vi "Save Instance VI to Polymorphic.vi"(8 "error in (no error)":errorcluster, 9 "Polymorphic Label":string, 10 "SubVI Ref In":refnum<vi>, 11 "Library Ref In":refnum<vi>) -> (0 "error out":errorcluster)   [LabVIEW 2020]
doc: "Duplicates the malleable VI instance to a new VI, and adds the new VI to a polymorphic VI."
uses:
  Global.vi
  <vilib>/LabVIEW Icon API/LabVIEW Icon API.lvlib
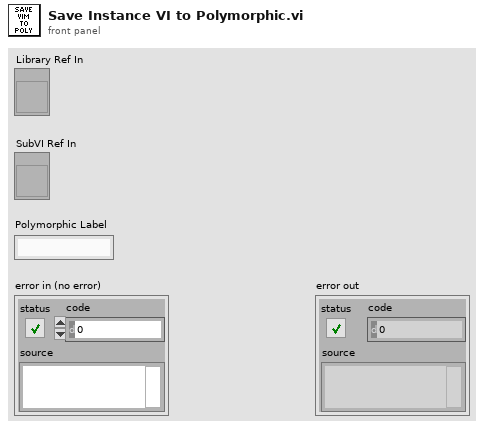
[diagram p1: front panel]
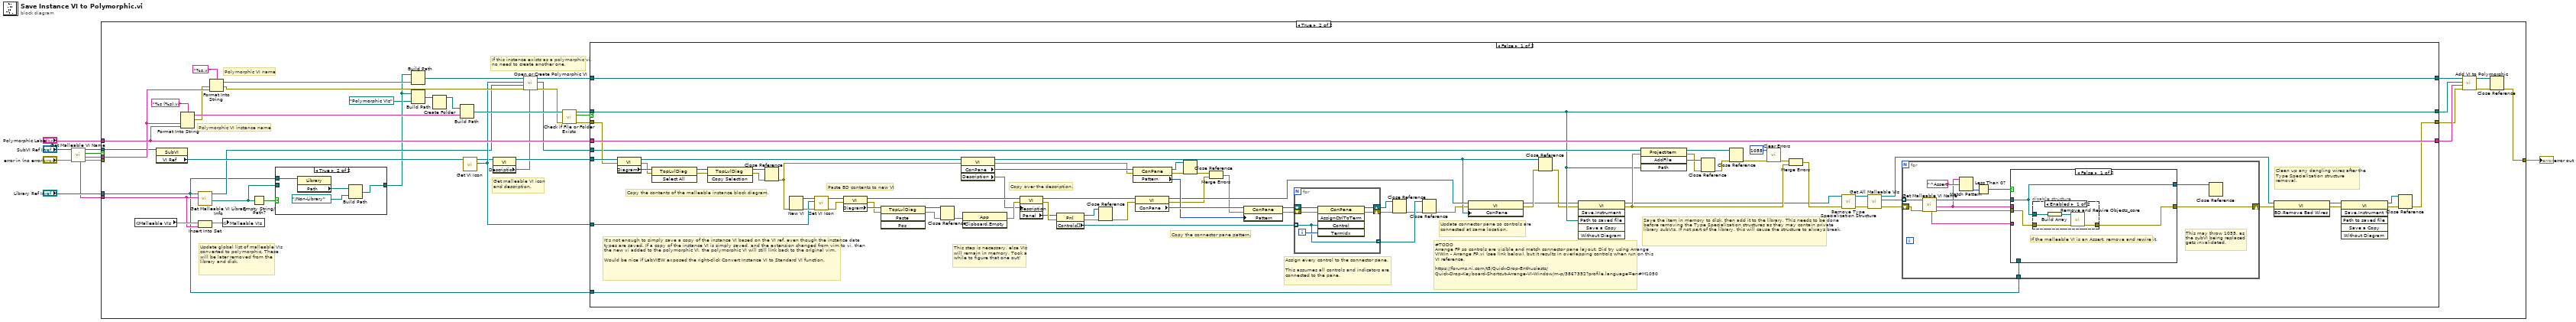
[diagram p0: block diagram]
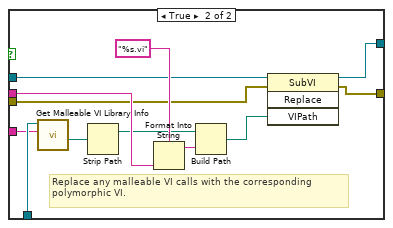
[diagram p4: hidden frame]
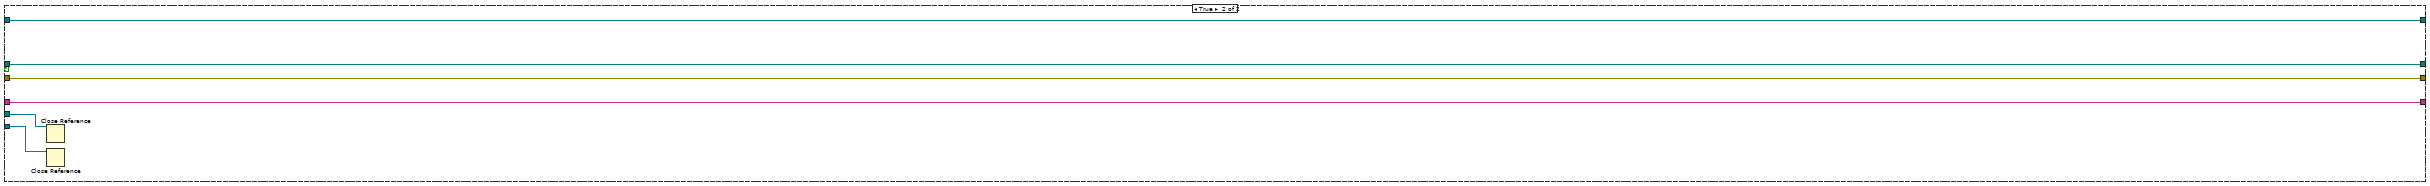
[diagram p5: hidden frame]
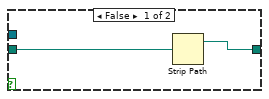
[diagram p6: hidden frame]
diagram:
  n1 = call "Get Malleable VI Name.vi"("error in (no error)"="error in (no error)", "SubVI Ref In"="SubVI Ref In") -> ("error out"=w5:errorcluster, "Name without extension"=w8:string, "Is Malleable VI?"=w1:bool, "SubVI Ref Out"=w9:refnum<vi>, "Name (unmodified)"=w2:string)  [unwired: 5 in]
  n2 = case shown="True" w1 {
    tunnel: w9 -> [_ w32]
    tunnel: w8 -> [_ w46]
    tunnel: "Polymorphic Label" -> [_ w48]
    tunnel: w5 -> [w11 _]
    tunnel: [w11 w33] -> w4
    tunnel: "Library Ref In" -> [_ w17]
    tunnel: w2 -> [_ w23]
    frame False {
    }
    frame True {
      # "Get malleable VI icon and description."
      # "Update global list of malleable VIs converted to polymorphic. These will be later removed from the library and disk."
      # "Polymorphic VI instance name"
      # "Polymorphic VI name"
      # "If this instance exists as a polymorphic vi, no need to create another one."
      n3 = global read "Global.vi" "Malleable VIs"() -> (w24:set{string})
      n4 = property on="Property Node" class="SubVI"(reference=w32) -> ("VI Ref"=w29:refnum<vi>)  [unwired: 1 in, 2 out]
      n5 = Format Into String(format string="%s (%s).vi", w46, w48) -> (resulting string=w51:string, error out=w38:errorcluster)  [unwired: 2 in]
      n6 = call "Get Malleable VI Library Info.vi"("Malleable VI Name"=w23, "Library Ref"=w17) -> ("Malleable VI Path"=w27:path, "Owner"=w28:refnum<vi>)  [unwired: 6 in, 2 out]
      n7 = Insert Into Set(10:w23, 11:w24) -> (3:w22:set{string})  [unwired: 1 out]
      n8 = Format Into String(format string="%s.vi", error in=w38, w46) -> (resulting string=w44:string, error out=w37:errorcluster)  [unwired: 1 in]
      n9 = global write "Global.vi" "Malleable VIs"(w22) -> ()
      n10 = Empty String/Path?(string/path=w27) -> (empty?=w30:bool)
      n11 = case shown="True" w30 {
        tunnel: w27 -> [w174 _]
        tunnel: [w173 w175] -> w15
        tunnel: w17 -> [_ w178]
        frame False {
          n12 = Strip Path(path=w174) -> (stripped path=w173:path)  [unwired: 1 out]
        }
        frame True {
          n13 = property on="Property Node" class="Library"(reference=w178) -> ("Path"=w177:path)  [unwired: 1 in, 2 out]
          n14 = Build Path(base path=w177, name or relative path=path "../Non-Library") -> (appended path=w175:path)
        }
      }
      n15 = Build Path(base path=w15, name or relative path=w44) -> (appended path=w43:path)
      n16 = Build Path(base path=w15, name or relative path=path "Polymorphic VIs") -> (appended path=w13:path)
      n17 = Create Folder(path (use dialog)=w13) -> (created path=w12:path)  [unwired: 2 in, 2 out]
      n18 = Build Path(base path=w12, name or relative path=w51) -> (appended path=w50:path)
      n19 = call <vilib>:"Get VI Icon.vi"("VI Refnum in"=w29) -> ("Icon"=w31:refnum<class "Icon.lvclass">, "VI Refnum out"=w20:refnum<vi>)  [unwired: 8 in, 1 out]
      n20 = property on="Property Node" class="VI"(reference=w20) -> (reference out=w19:refnum<vi>, "Description"=w18:string)  [unwired: 1 in, 1 out]
      n21 = call "Open or Create Polymorphic VI.vi"("Description"=w18, "error in (no error)"=w37, "Owner"=w28, "Icon"=w31, "Polymorphic VI Path In"=w43) -> ("error out"=w36:errorcluster, "Polymorphic Library Owner"=w16:refnum<vi>, "Polymorphic VI Refnum"=w42:refnum<vi>)  [unwired: 4 in]
      n22 = call <vilib>:"Check if File or Folder Exists.vi"("error in (no error)"=w36, "path"=w50) -> ("error out"=w35:errorcluster, "file or folder exists?"=w21:bool, "dup path"=w49:path)  [unwired: 7 in]
      n23 = case shown="False" w21 {
        tunnel: w49 -> [w65 w171]
        tunnel: w48 -> [w105 w170]
        tunnel: w42 -> [w106 w172]
        tunnel: [w106 w172] -> w41
        tunnel: [w65 w171] -> w40
        tunnel: [w105 w170] -> w39
        tunnel: w35 -> [w103 w169]
        tunnel: [w73 w169] -> w34
        tunnel: w19 -> [w104 w167]
        tunnel: w31 -> [w98 _]
        tunnel: w16 -> [w80 w168]
        tunnel: w17 -> [w56 _]
        frame False {
          # "#TODO\nArrange FP so controls are visible and match connector pane layout. Did try using Arrange VIWin - Arrange FP.vi (see link below), but it results in overlapping controls when run on this VI reference.\n\nhttps://forums.ni.com/t5/Quick-Drop-Enthusiasts/Quick-Drop-Keyboard-Shortcut-Arrange-VI-Window/m-p/3867352?profile.language=en#M1050"
          # "Clean up any dangling wires after the Type Specialization structure removal."
          # "Update connector pane so controls are connected at same location."
          # "Copy the connector pane pattern."
          # "Assign every control to the connector pane.\n\nThis assumes all controls and indicators are connected to the pane."
          # "Copy over the description."
          # "Paste BD contents to new VI"
          # "This step is necessary, else VIs will remain in memory. Took a while to figure that one out!"
          # "Save the item in memory to disk, then add it to the library. This needs to be done before removing the Type Specialization structures as they may contain private library subVIs. If not part of the library, this will cause the structure to always break."
          # "It's not enough to simply save a copy of the instance VI based on the VI ref, even though the instance data types are saved. If a copy of the instance VI is simply saved, and the extension changed from vim to vi, then the new vi added to the polymorphic VI, the polymorphic VI will still link back to the original vim.\n\nWould be nice if LabVIEW exposed the right-click Convert Instance VI to Standard VI function."
          # "Copy the contents of the malleable instance block diagram."
          n24 = property on="Property Node" class="VI"(reference=w104, error in=w103) -> (reference out=w117:refnum<vi>, error out=w125:errorcluster, "Diagram"=w128:refnum<vi>)
          n25 = invoke on="Invoke Node" class="TopLvlDiag" method="Select All"(reference=w128, error in=w125) -> (reference out=w127:refnum<vi>, error out=w124:errorcluster)  [unwired: 1 in, 1 out]
          n26 = invoke on="Invoke Node" class="TopLvlDiag" method="Copy Selection"(reference=w127, error in=w124) -> (reference out=w110:refnum<vi>, error out=w109:errorcluster)  [unwired: 1 in, 1 out]
          n27 = Close Reference(reference=w110, error in (no error)=w109) -> (error out=w108:errorcluster)
          n28 = New VI(8:w108) -> (0:w100:errorcluster, 3:w102:refnum<vi>)  [unwired: 6 in]
          n29 = call <vilib>:"Set VI Icon.vi"("error in (no error)"=w100, "Icon"=w98, "VI Refnum in"=w102) -> ("error out"=w99:errorcluster, "VI Refnum out"=w101:refnum<vi>)  [unwired: 7 in]
          n30 = property on="Property Node" class="VI"(reference=w101, error in=w99) -> (reference out=w122:refnum<vi>, error out=w123:errorcluster, "Diagram"=w126:refnum<vi>)
          n31 = invoke on="Invoke Node" class="TopLvlDiag" method="Paste"(reference=w126, error in=w123) -> (reference out=w90:refnum<vi>, error out=w91:errorcluster)  [unwired: 2 in, 2 out]
          n32 = Close Reference(reference=w90, error in (no error)=w91) -> (error out=w69:errorcluster)
          n33 = property on="Property Node" class="VI"(reference=w117, error in=w108) -> (reference out=w81:refnum<vi>, error out=w107:errorcluster, "ConPane"=w118:refnum<vi>, "Description"=w67:string)
          n34 = invoke on="Invoke Node" class="App" method="Clipboard.Empty"(error in=w69) -> (error out=w68:errorcluster)  [unwired: 2 in, 2 out]
          n35 = property on="Property Node" class="VI"(reference=w122, error in=w68, "Description"=w67) -> (reference out=w120:refnum<vi>, error out=w121:errorcluster, "Panel"=w111:refnum<vi>)
          n36 = property on="Property Node" class="Pnl"(reference=w111, error in=w121) -> (reference out=w89:refnum<vi>, error out=w88:errorcluster, "Controls[]"=w114:refnum<vi>[])
          n37 = Close Reference(reference=w89, error in (no error)=w88) -> (error out=w87:errorcluster)
          n38 = property on="Property Node" class="ConPane"(reference=w118, error in=w107) -> (reference out=w86:refnum<vi>, error out=w85:errorcluster, "Pattern"=w116:u32)
          n39 = property on="Property Node" class="VI"(reference=w120, error in=w87) -> (reference out=w113:refnum<vi>, error out=w97:errorcluster, "ConPane"=w119:refnum<vi>)
          n40 = Close Reference(reference=w86, error in (no error)=w85) -> (error out=w84:errorcluster)
          n41 = Merge Errors(w84, w97) -> (w96:errorcluster)
          n42 = property on="Property Node" class="ConPane"(reference=w119, error in=w96, "Pattern"=w116) -> (reference out=w115:refnum<vi>, error out=w112:errorcluster)
          n43 = for {
            tunnel: w114 -> [w161] mode=indexing
            shift-right: [w164] -> w83
            shift-left: w115 -> [w166]
            shift-right: [w162] -> w82
            shift-left: w112 -> [w163]
            tunnel: [w161] -> w72 mode=indexing
            i -> [w165]
            n44 = invoke on="Invoke Node" class="ConPane" method="AssignCtrlToTerm"(reference=w166, error in=w163, "Control"=w161, "TermIdx"=w165) -> (reference out=w164:refnum<vi>, error out=w162:errorcluster)  [unwired: 1 in, 3 out]
          }
          n45 = Close Reference(reference=w83, error in (no error)=w82) -> (error out=w71:errorcluster)
          n46 = Close Reference(reference=w72, error in (no error)=w71) -> (error out=w70:errorcluster)
          n47 = property on="Property Node" class="VI"(reference=w113, error in=w70, "ConPane"=w81) -> (reference out=w64:refnum<vi>, error out=w66:errorcluster)
          n48 = Close Reference(reference=w81, error in (no error)=w66) -> (error out=w63:errorcluster)
          n49 = invoke on="Invoke Node" class="VI" method="Save.Instrument"(reference=w64, error in=w63, "Path to saved file"=w65) -> (reference out=w57:refnum<vi>, error out=w76:errorcluster)  [unwired: 3 in, 4 out]
          n50 = invoke on="Invoke Node" class="ProjectItem" method="AddFile"(reference=w80, error in=w76, "Path"=w65) -> (reference out=w93:refnum<vi>, error out=w78:errorcluster, "AddFile"=w79:refnum<vi>)  [unwired: 1 in, 1 out]
          n51 = Close Reference(reference=w79, error in (no error)=w78) -> (error out=w77:errorcluster)
          n52 = Close Reference(reference=w93, error in (no error)=w77) -> (error out=w92:errorcluster)
          n53 = call <vilib>:"Clear Errors.vi"("error in (no error)"=w92, "specific error code to clear (0: all)"=1055) -> ("error out"=w94:errorcluster)  [unwired: 4 in, 1 out]
          n54 = Merge Errors(w94, w76) -> (w58:errorcluster)
          n55 = call "Remove Type Specialization Structure.vi"("error in (no error)"=w58, "VI Ref In"=w57) -> ("error out"=w60:errorcluster, "VI Ref Out"=w59:refnum<vi>)  [unwired: 8 in]
          n56 = call "Get All Malleable VIs.vi"("error in (no error)"=w60, "VI Ref In"=w59) -> ("error out"=w61:errorcluster, "Malleable VIs"=w62:refnum<vi>[], "VI Ref Out"=w55:refnum<vi>)  [unwired: 7 in]
          n57 = for {
            tunnel: w62 -> [w140] mode=indexing
            shift-right: [w134] -> w53
            shift-left: w61 -> [w138]
            tunnel: w56 -> [w136]
            # "This may throw 1055, as the subVI being replaced gets invalidated."
            n58 = call "Get Malleable VI Name.vi"("error in (no error)"=w138, "SubVI Ref In"=w140) -> ("error out"=w137:errorcluster, "Name without extension"=w131:string, "SubVI Ref Out"=w139:refnum<vi>, "Name (unmodified)"=w135:string)  [unwired: 5 in, 1 out]
            n59 = Match Pattern(string=w131, regular expression="^Assert") -> (offset past match=w132:i32)  [unwired: 1 in, 3 out]
            n60 = Less Than 0?(x=w132) -> (x < 0?=w129:bool)
            n61 = case shown="False" w129 {
              tunnel: w131 -> [_ w160]
              tunnel: w139 -> [w143 w157]
              tunnel: w137 -> [w142 w155]
              tunnel: w136 -> [_ w154]
              tunnel: w135 -> [_ w153]
              tunnel: [w141 w150] -> w134
              tunnel: [w143 w149] -> w130
              frame False {
                # "If the malleable VI is an Assert, remove and rewire it."
                n62 = disable-structure "Diagram Disable Structure" shown="Enabled" {
                  disable-tunnel: w143 -> [w146 _]
                  disable-tunnel: w142 -> [w145 w148]
                  disable-tunnel: [w144 w148] -> w141
                  frame Enabled {
                    n63 = Build Array(w146) -> (w147:refnum<vi>[])
                    n64 = call <vilib>:"Remove and Rewire Objects_core.vi"("error in (no error)"=w145, "Items to Remove"=w147) -> ("error out"=w144:errorcluster)  [unwired: 8 in, 1 out]
                  }
                  frame Disabled {
                  }
                }
              }
              frame True {
                # "Replace any malleable VI calls with the corresponding polymorphic VI."
                n65 = call "Get Malleable VI Library Info.vi"("Malleable VI Name"=w153, "Library Ref"=w154) -> ("Malleable VI Path"=w152:path)  [unwired: 6 in, 3 out]
                n66 = Strip Path(path=w152) -> (stripped path=w151:path)  [unwired: 1 out]
                n67 = Format Into String(format string="%s.vi", w160) -> (resulting string=w158:string)  [unwired: 2 in, 1 out]
                n68 = Build Path(base path=w151, name or relative path=w158) -> (appended path=w156:path)
                n69 = invoke on="Invoke Node" class="SubVI" method="Replace"(reference=w157, error in=w155, "VIPath"=w156) -> (reference out=w149:refnum<vi>, error out=w150:errorcluster)  [unwired: 1 in, 2 out]
              }
            }
            n70 = Close Reference(reference=w130) -> ()  [unwired: 1 in, 1 out]
          }
          n71 = invoke on="Invoke Node" class="VI" method="BD.Remove Bad Wires"(reference=w55, error in=w53) -> (reference out=w54:refnum<vi>, error out=w52:errorcluster)  [unwired: 1 in, 1 out]
          n72 = invoke on="Invoke Node" class="VI" method="Save.Instrument"(reference=w54, error in=w52) -> (reference out=w75:refnum<vi>, error out=w74:errorcluster)  [unwired: 4 in, 4 out]
          n73 = Close Reference(reference=w75, error in (no error)=w74) -> (error out=w73:errorcluster)
        }
        frame True {
          n74 = Close Reference(reference=w168) -> ()  [unwired: 1 in, 1 out]
          n75 = Close Reference(reference=w167) -> ()  [unwired: 1 in, 1 out]
        }
      }
      n76 = call "Add VI to Polymorphic.vi"("error in (no error)"=w34, "Polymorphic Label"=w39, "Path"=w40, "Polymorphic VI Refnum In"=w41) -> ("error out"=w25:errorcluster, "Polymorphic VI Refnum Out"=w26:refnum<vi>)  [unwired: 6 in]
      n77 = Close Reference(reference=w26, error in (no error)=w25) -> (error out=w33:errorcluster)
    }
  }
  "error out" <- w4
